vi "movXY.vi"(0 "y pos (mm)":dbl, 1 "x pos (mm)":dbl, 2 "xy cluster":T1) -> ()   [LabVIEW 2015]
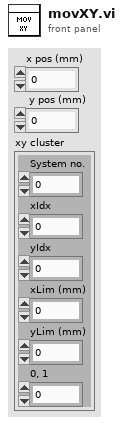
[diagram p1: front panel]
types:
  T1 = cluster{"System no.":i32, "xIdx":i32, "yIdx":i32, "xLim (mm)":dbl, "yLim (mm)":dbl, "0, 1":i16}
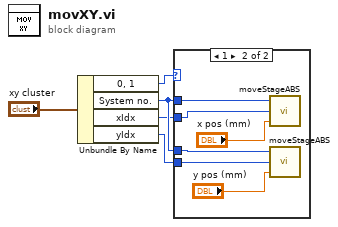
[diagram p0: block diagram]
diagram:
  n1 = Unbundle By Name("xy cluster") -> ("0, 1"=w5:i16, "System no."=w4:i32, "xIdx"=w3:i32, "yIdx"=w2:i32)
  n2 = case shown="1" w5 {
    tunnel: w4 -> [_ w11]
    tunnel: w4 -> [_ w10]
    tunnel: w3 -> [_ w9]
    tunnel: w2 -> [_ w8]
    frame 0, Default {
    }
    frame 1 {
      n3 = call "moveStageABS.vi"("absolute pos (mm)"="x pos (mm)", "axisIdx"=w9, "System no."=w11) -> ()  [unwired: 1 out]
      n4 = call "moveStageABS.vi"("absolute pos (mm)"="y pos (mm)", "axisIdx"=w8, "System no."=w10) -> ()  [unwired: 1 out]
    }
  }
